vi "Calculate switching matrix.vi"(9 "Ch. bytes 2":u8[](array[numeric]), 10 "Ch. bytes 1":u8[](array[numeric])) -> (2 "Array":bool[][](array[boolean]))   [LabVIEW 2020, in "QuPMXdriver.lvlib"]
doc: "Converts bytes to switching sequence (array of channel states)."
uses:
  QuPMXdriver.lvlib
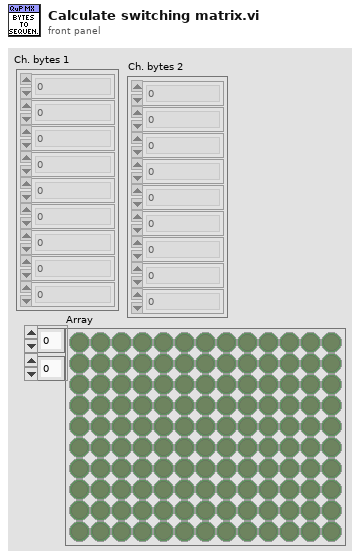
[diagram p1: front panel]
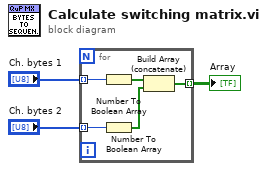
[diagram p0: block diagram]
diagram:
  n1 = for {
    tunnel: "Ch. bytes 1" -> [w8] mode=indexing
    tunnel: "Ch. bytes 2" -> [w7] mode=indexing
    tunnel: [w4] -> w1 mode=indexing
    n2 = Number To Boolean Array(number=w8) -> (Boolean array=w6:bool[])
    n3 = Number To Boolean Array(number=w7) -> (Boolean array=w5:bool[])
    n4 = Build Array (concatenate)(w6, w5) -> (w4:bool[])
  }
  "Array" <- w1
